vi "Command Drive Distance with Heading Delay.vi"(8 "Segments":dbl=18.0, 9 "Heading":dbl, 10 "Distance":dbl=90.0, 11 "Startup":bool) -> (0 "Right Wheel":dbl=nan, 1 "Reinit":bool, 2 "Left Wheel":dbl=-2723.84, 3 "Completed":bool)   [LabVIEW 2019]
uses:
  Drive/Drive Globals.vi
  Utility VIs/Refnum Names.vi
panel:
  out "Waveform Chart":dbl(graph)
  out "Distance Increment":dbl
  out "Heading Increment":dbl
  out "Initial Heading":dbl=56.4697265625
  in  "Turn Gain":dbl=0.06
  in  "Gain":dbl=0.028
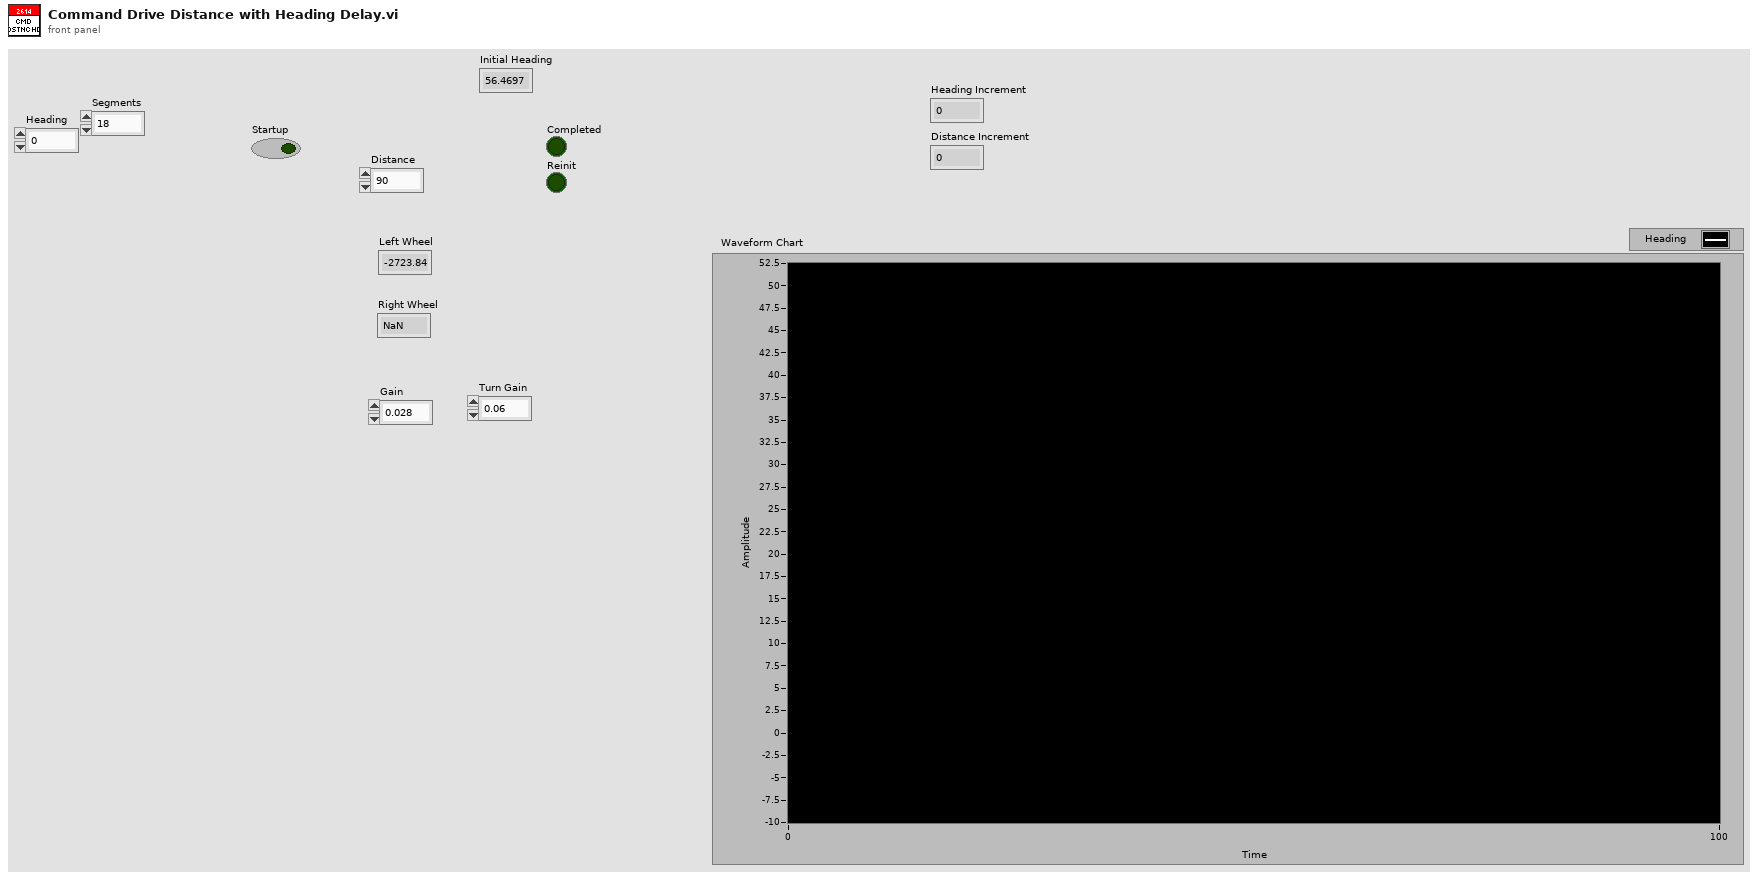
[diagram p1: front panel]
types:
  T1 = typedef "WPI_MotorControlDeviceRef.ctl" = cluster{"DeviceStatus":errorcluster, "Type":T2, "PWM":cluster{"PWM Channel":T3, "DeadBand":T4}, "CAN":cluster{"Device Number":u8, "SetOutput VI Ref":variant, "GetOutput VI Ref":variant, "Enable VI Ref":variant, "Disable VI Ref":variant, "Data":variant}, "Invert":bool, "DIO PWM":cluster{"PWM \"Enable\" Channel":T3, "DIOChannel":T5, "PWM Rate":dbl}}
  T2 = typedef "WPI_MotorControlType.ctl" = enum16{"PWM", "CAN", "DIO PWM"}
  T3 = typedef "FPGA_DIOPWMChannel.ctl" = enum8{"PWM 0", "PWM 1", "PWM 2", "PWM 3", "PWM 4", "PWM 5", "PWM 6", "PWM 7", "PWM 8", "PWM 9", "PWM MXP 0", "PWM MXP 1", "PWM MXP 2", "PWM MXP 3", "PWM MXP 4", "PWM MXP 5", "PWM MXP 6", "PWM MXP 7", "PWM MXP 8", "PWM MXP 9", "Invalid"}
  T4 = typedef "WPI_PWMDeadband.ctl" = cluster{"Name":string, "maxPositivePwm":i32, "minPositivePwm":i32, "centerPwm":i32, "maxNegativePwm":i32, "minNegativePwm":i32, "angularRange":u16}
  T5 = typedef "FPGA_DIOChannel.ctl" = enum8{"DIO 0", "DIO 1", "DIO 2", "DIO 3", "DIO 4", "DIO 5", "DIO 6", "DIO 7", "DIO 8", "DIO 9", "DIO MXP 0", "DIO MXP 1", "DIO MXP 2", "DIO MXP 3", "DIO MXP 4", "DIO MXP 5", "DIO MXP 6", "DIO MXP 7", "DIO MXP 8", "DIO MXP 9", "DIO MXP 10", "DIO MXP 11", "DIO MXP 12", "DIO MXP 13", "DIO MXP 14", "DIO MXP 15", "SPI Port CS1", "SPI Port CS2", "SPI Port CS3", "SPI Port MISO", "SPI Port MOSI", "Invalid"}
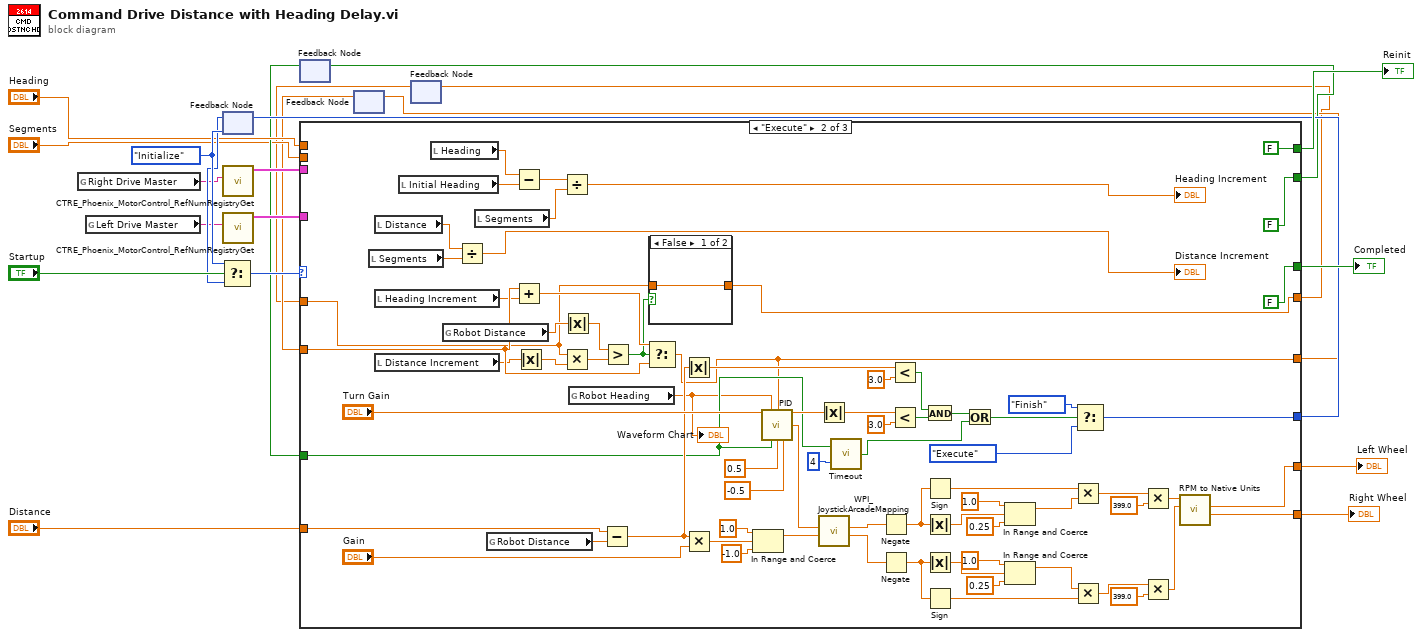
[diagram p0: block diagram]
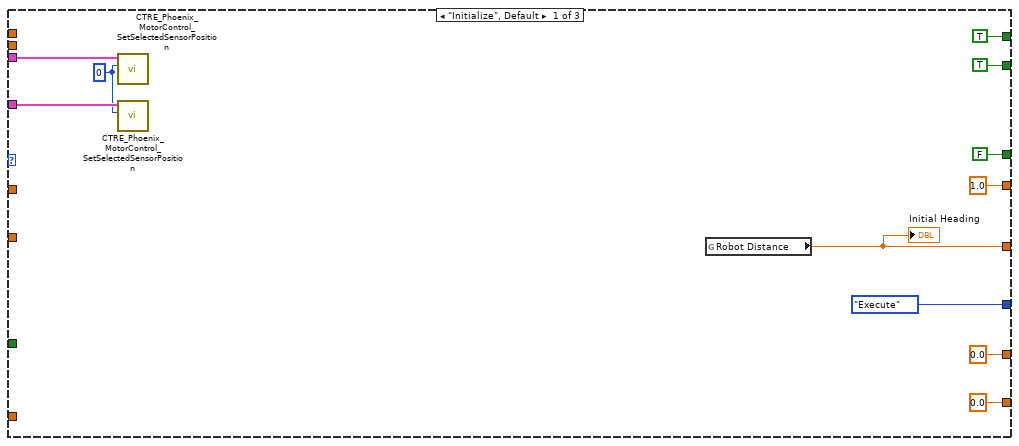
[diagram p2: hidden frame]
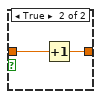
[diagram p3: hidden frame]
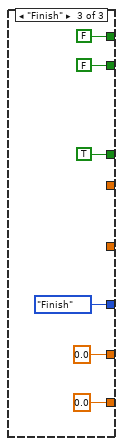
[diagram p4: hidden frame]
diagram:
  w20 = enum16{"Initialize", "Execute", "Finish"}."Initialize"
  n1 = global read "Refnum Names.vi" "Right Drive Master"() -> (w11:string)
  n2 = global read "Refnum Names.vi" "Left Drive Master"() -> (w12:string)
  n3 = feedback #1(w20) -> (w16:enum16{"Initialize", "Execute", "Finish"})
  n4 = Select(t=w20, s="Startup", f=w16) -> (s? t:f=w21:enum16{"Initialize", "Execute", "Finish"})
  n5 = call <vilib>:"CTRE_Phoenix_MotorControl_RefNumRegistryGet.vi"("refnum name"=w11) -> ("PhoenixMotorControlDevRef"=w10:T1)  [unwired: 9 in, 1 out]
  n6 = call <vilib>:"CTRE_Phoenix_MotorControl_RefNumRegistryGet.vi"("refnum name"=w12) -> ("PhoenixMotorControlDevRef"=w9:T1)  [unwired: 9 in, 1 out]
  n7 = feedback #2() -> (w6:bool)  [unwired: 1 in]
  n8 = feedback #3() -> (w3:dbl)  [unwired: 1 in]
  n9 = feedback #4() -> (w1:dbl)  [unwired: 1 in]
  n10 = case shown="\"Execute\"" w21 {
    tunnel: [FALSE FALSE TRUE] -> w19
    tunnel: [TRUE FALSE FALSE] -> w18
    tunnel: [enum16{"Initialize", "Execute", "Finish"}."Execute" w103 enum16{"Initialize", "Execute", "Finish"}."Finish"] -> w17
    tunnel: "Distance" -> [_ w59 _]
    tunnel: [0.0 ("Left Wheel Velocity") w63 0.0] -> w14
    tunnel: [0.0 ("Right Wheel Velocity") w62 0.0] -> w13
    tunnel: w10 -> [w27 _ _]
    tunnel: w9 -> [w28 _ _]
    tunnel: "Heading" -> [_ _ _]
    tunnel: [TRUE FALSE FALSE] -> w7
    tunnel: w6 -> [_ w58 _]
    tunnel: "Segments" -> [_ _ _]
    tunnel: [w24 w53 _] -> w4
    tunnel: w3 -> [_ w54 _]
    tunnel: [1.0 ("Left Wheel Velocity") w36 _] -> w2
    tunnel: w1 -> [_ w35 _]
    frame "Initialize", Default {
      w26 = 0
      n11 = call <vilib>:"CTRE_Phoenix_MotorControl_SetSelectedSensorPosition.vi"("New Sensor Position"=w26, "PhoenixMotorControlDevRef"=w27) -> ()  [unwired: 8 in, 2 out]
      n12 = call <vilib>:"CTRE_Phoenix_MotorControl_SetSelectedSensorPosition.vi"("New Sensor Position"=w26, "PhoenixMotorControlDevRef"=w28) -> ()  [unwired: 8 in, 2 out]
      n13 = global read "Drive Globals.vi" "Robot Distance"() -> (w24:dbl)
      "Initial Heading" <- w24
    }
    frame "Execute" {
      n14 = local read "Segments"() -> (w42:dbl)
      n15 = local read "Distance"() -> (w43:dbl)
      n16 = local read "Heading Increment"() -> (w44:dbl)
      n17 = local read "Distance Increment"() -> (w47:dbl)
      n18 = local read "Initial Heading"() -> (w51:dbl)
      n19 = local read "Heading"() -> (w52:dbl)
      n20 = global read "Drive Globals.vi" "Robot Distance"() -> (w40:dbl)
      n21 = Divide(x=w43, y=w42) -> (x/y=→"Distance Increment":dbl)
      n22 = local read "Segments"() -> (w50:dbl)
      n23 = global read "Drive Globals.vi" "Robot Distance"() -> (w55:dbl)
      n24 = Subtract(x=w52, y=w51) -> (x-y=w49:dbl)
      n25 = Add(x=w54, y=w44) -> (x+y=w46:dbl)
      n26 = Absolute Value(x=w47) -> (abs(x)=w45:dbl)
      n27 = Divide(x=w49, y=w50) -> (x/y=→"Heading Increment":dbl)
      n28 = Multiply(x=w35, y=w45) -> (x*y=w38:dbl)
      n29 = Absolute Value(x=w40) -> (abs(x)=w39:dbl)
      n30 = global read "Drive Globals.vi" "Robot Heading"() -> (w34:dbl)
      "Waveform Chart" <- w34
      n31 = Subtract(x=w59, y=w55) -> (x-y=w60:dbl)
      n32 = Greater?(x=w39, y=w38) -> (0:w37:bool)
      n33 = Select(t=w46, s=w37, f=w54) -> (s? t:f=w53:dbl)
      n34 = case shown="False" w37 {
        tunnel: [w107 w109] -> w36
        tunnel: w35 -> [w107 w108]
        frame False {
        }
        frame True {
          n35 = Increment(x=w108) -> (x+1=w109:dbl)
        }
      }
      n36 = Absolute Value(x=w60) -> (abs(x)=w101:dbl)
      n37 = Multiply(x=w60, y="Gain") -> (x*y=w98:dbl)
      n38 = In Range and Coerce(upper limit=1.0, x=w98, lower limit=-1.0) -> (coerced(x)=w87:dbl)  [unwired: 1 out]
      n39 = call "PID.vi"("Kp"="Turn Gain", "Process Variable"=w34, "Goal"=w53, "Reinit"=w58, "Max Ouput"=0.5, "Min Output"=-0.5) -> ("Current Error"=w89:dbl, "Command"=w88:dbl)  [unwired: 7 in, 1 out]
      n40 = Absolute Value(x=w89) -> (abs(x)=w91:dbl)
      n41 = call <vilib>:"WPI_JoystickArcadeMapping.vi"("Y axis value"=w87, "X axis value"=w88) -> ("Right Motor Value"=w85:dbl, "Left Motor Value"=w86:dbl)  [unwired: 8 in]
      n42 = call "Timeout.vi"("Timeout"=u32 4, "Initialize"=w58) -> ("Timed Out?"=w80:bool)
      n43 = Negate(x=w86) -> (-x=w76:dbl)
      n44 = Negate(x=w85) -> (-x=w77:dbl)
      n45 = Less?(x=w101, y=3.0) -> (x < y?=w93:bool)
      n46 = Less?(x=w91, y=3.0) -> (x < y?=w90:bool)
      n47 = And(x=w93, y=w90) -> (x .and. y?=w94:bool)
      n48 = Sign(1:w76) -> (0:w75:dbl)
      n49 = Absolute Value(x=w76) -> (abs(x)=w79:dbl)
      n50 = Absolute Value(x=w77) -> (abs(x)=w78:dbl)
      n51 = Sign(1:w77) -> (0:w70:dbl)
      n52 = Or(x=w94, y=w80) -> (x .or. y?=w81:bool)
      n53 = In Range and Coerce(upper limit=1.0, x=w79, lower limit=0.25) -> (coerced(x)=w74:dbl)  [unwired: 1 out]
      n54 = In Range and Coerce(upper limit=1.0, x=w78, lower limit=0.25) -> (coerced(x)=w71:dbl)  [unwired: 1 out]
      n55 = Multiply(x=w75, y=w74) -> (x*y=w73:dbl)
      n56 = Multiply(x=w71, y=w70) -> (x*y=w72:dbl)
      n57 = Select(t=enum16{"Initialize", "Execute", "Finish"}."Finish", s=w81, f=enum16{"Initialize", "Execute", "Finish"}."Execute") -> (s? t:f=w103:enum16{"Initialize", "Execute", "Finish"})
      n58 = Multiply(x=w73, y=399.0) -> (x*y=w65:dbl)
      n59 = Multiply(x=w72, y=399.0) -> (x*y=w64:dbl)
      n60 = call "RPM to Native Units.vi"("Right RPM"=w64, "Left RPM"=w65) -> ("Right Out"=w62:dbl, "Left Out"=w63:dbl)  [unwired: 6 in, 1 out]
    }
    frame "Finish" {
    }
  }
  "Completed" <- w19
  "Reinit" <- w18
  "Left Wheel" <- w14
  "Right Wheel" <- w13
  n61 = feedback-in #1(w17) -> ()
  n62 = feedback-in #2(w7) -> ()
  n63 = feedback-in #3(w4) -> ()
  n64 = feedback-in #4(w2) -> ()
